vi "FileExplorerMain.vi"(0 "Top Level Folder Path":path, 4 "Tree":string[](tree), 5 "Search Bar":string, 7 "Copy":bool, 9 "Expand / Colapse":bool, 11 "error in (no error)":errorcluster) -> (6 "Report String":string, 15 "error out":errorcluster)   [LabVIEW 2023]
doc: "This VI is the demonstration of the File explorer using tree with options like search, copy, expand/collapse the tree items populated from the input file path."
uses:
  TypeDefs/FileExplorerQueueOperations.ctl
  TypeDefs/FileExplorerStateDataCluster.ctl
  TypeDefs/FileExplorerDataCluster.ctl
panel:
  # "INSTRUCTIONS\n\n1. Run the VI.\n2. Choose the any folder path using \"Top Level Folder Path\" Control.\n3. Tree is populated with the selected folder hierarchy.\n4. Press \"Expand/Collapse\" button to expand or collapse the Folders in the tree.\n5. Enter folder name in the \"Search Bar\" and press enter to expand on particular folder.\n6. Select any files in the tree and press \"Copy\" to copy the file to the desired location.\n7. Whenever a folder is expanded, particular folder details is indicated in the \"Report String\"\n8. Press the Column Headers to sort the tree based on the selection like Date Modified, Type or size"
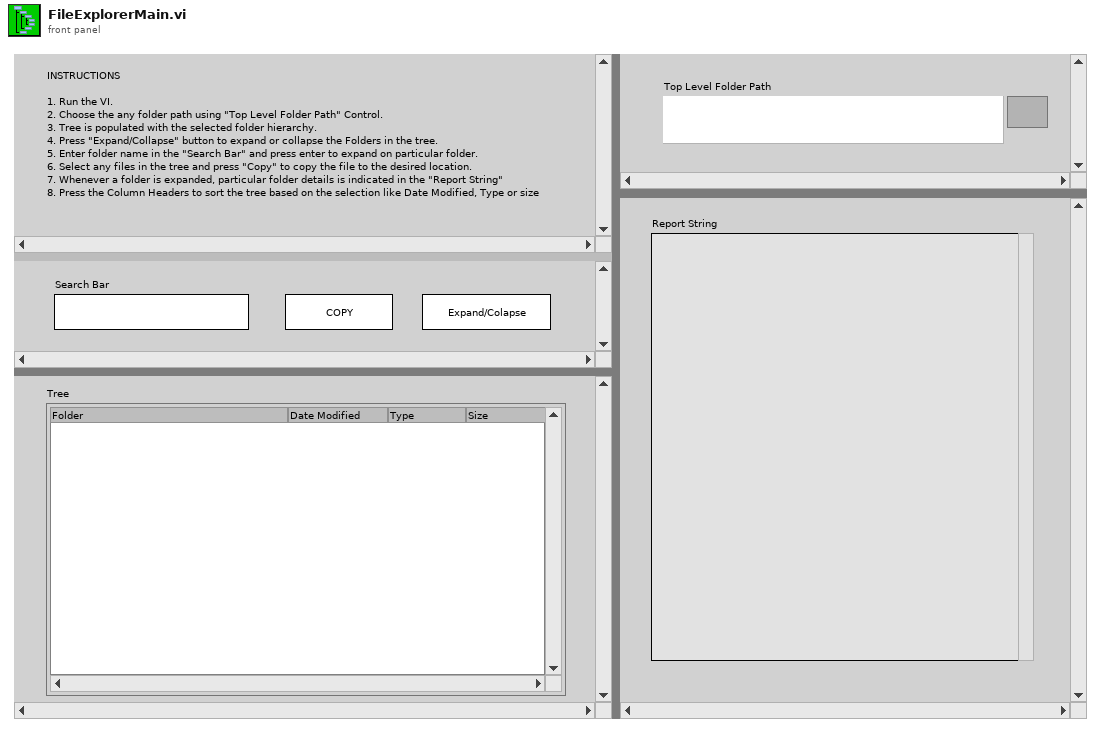
[diagram p1: front panel]
types:
  T1 = typedef "FileExplorerDataCluster.ctl" = cluster{"user event ref":refnum<user-event>, "Search Bar":string, "File Path":path, "All Folders Path":path[], "All Files Path":path[], "Parent Tag":string, "Reverse File Path":path, "End File":string[], "Tag Path":string[], "Selected file array":string[], "Tag Date Modified":string, "Tag Size":string, "Tag Type":string, "Report String":string, "Sort Date":bool, "Sort Type":bool, "Sort Size":bool, "Copied File Path array":path[], "Temp File Path":path, "Copy file Folder":string, "Active Tag":string, "Folders Array":string[]}
  T2 = typedef "FileExplorerStateDataCluster.ctl" = cluster{"State":string, "Data":variant}
  T3 = typedef "FileExplorerQueueOperations.ctl" = enum16{"Init", "Enqueue", "Dequeue", "Enqueue N", "Flush", "Close", "Enqueue N Stack"}
  T4 = typedef "LVPoint32TypeDef.ctl" = cluster{"Horizontal":i32, "Vertical":i32}
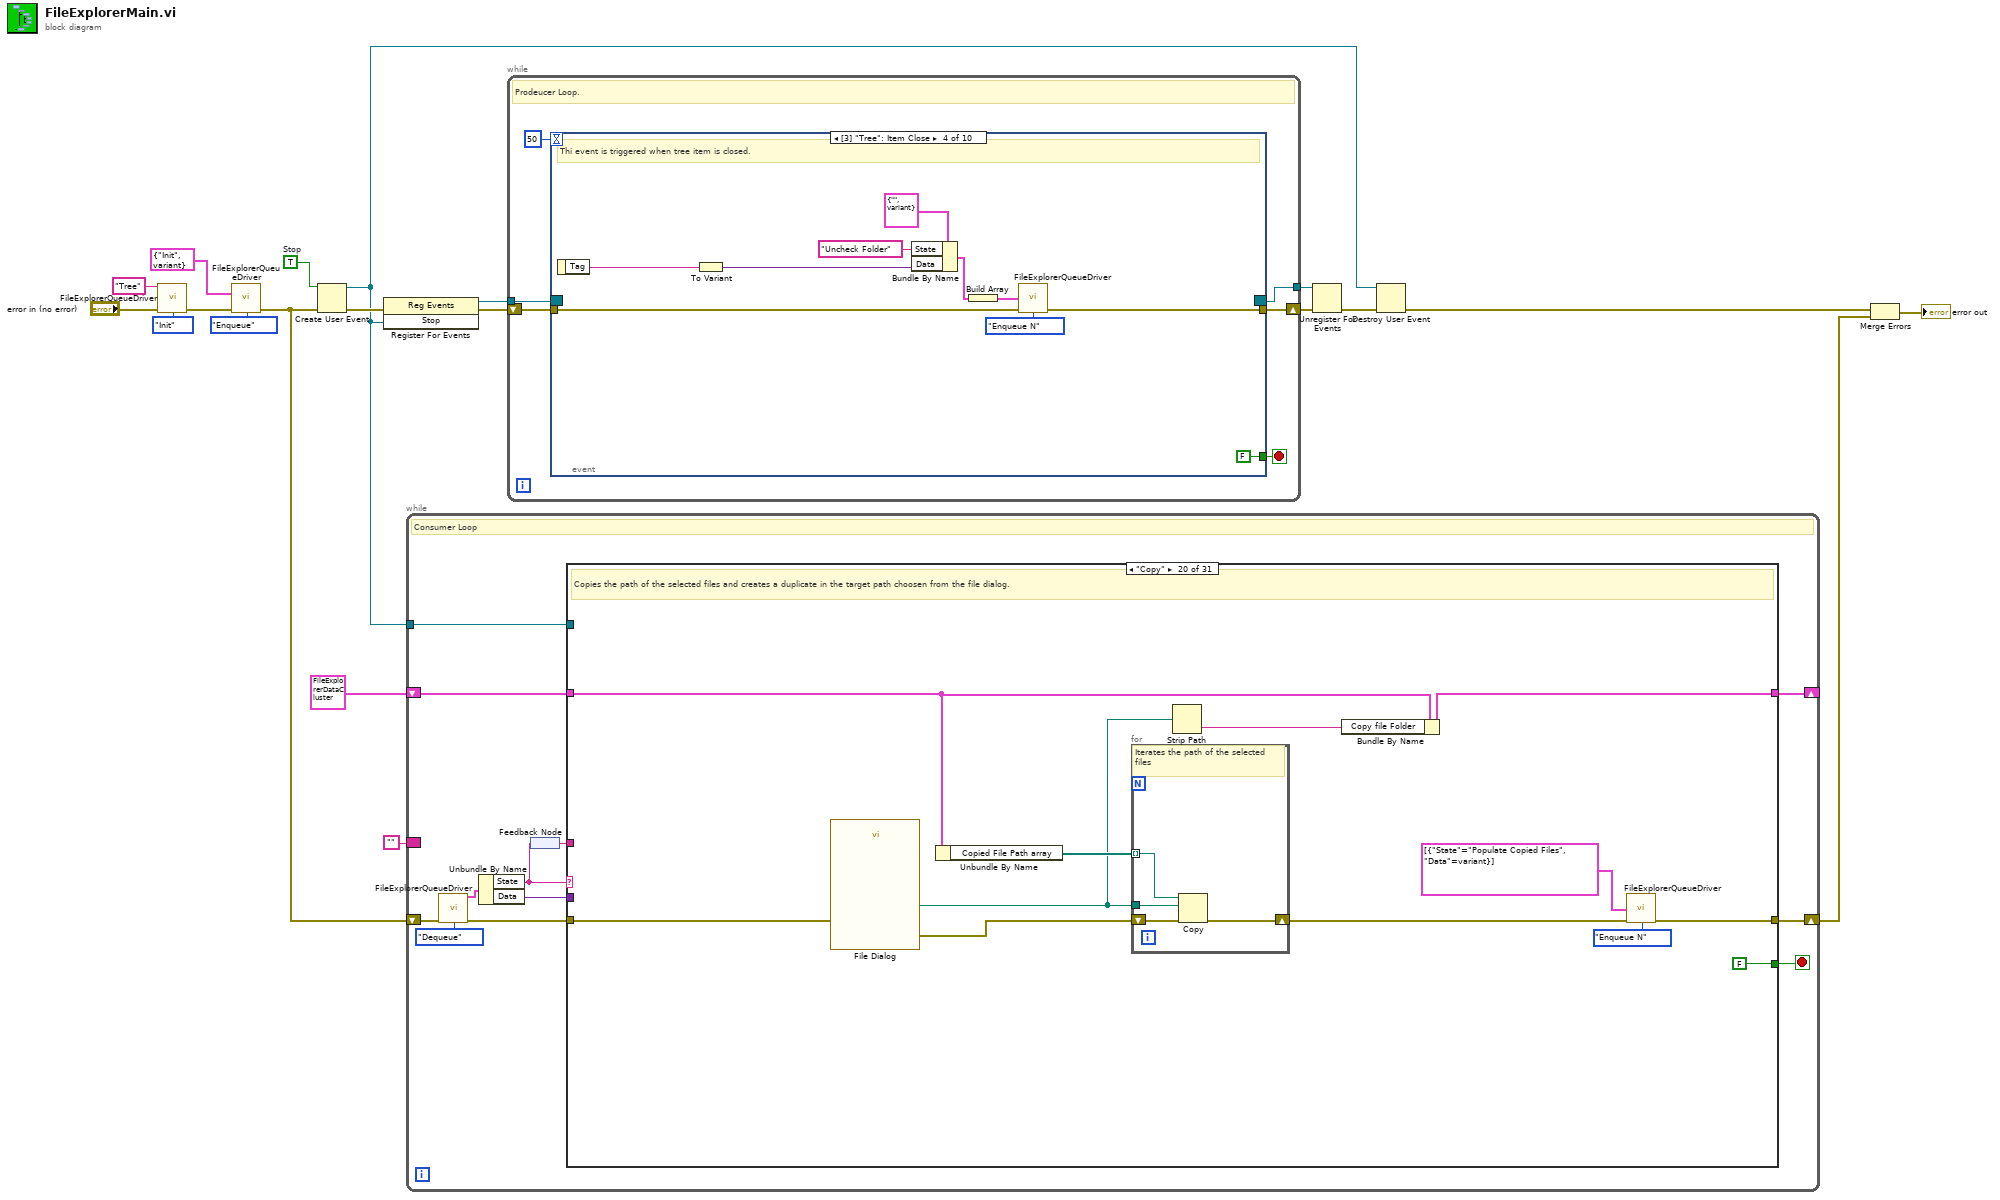
[diagram p0: block diagram]
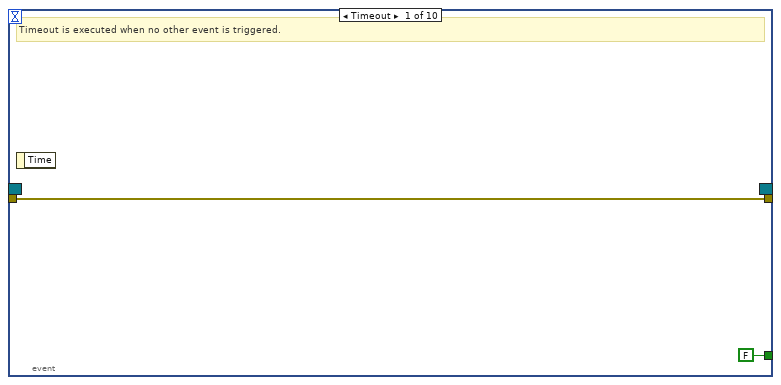
[diagram p2: hidden frame]
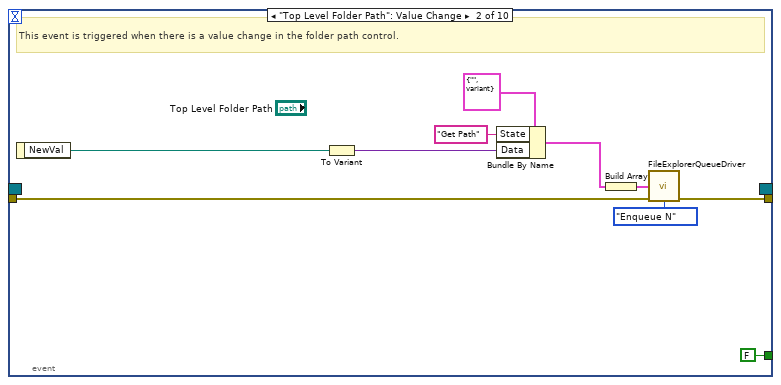
[diagram p3: hidden frame]
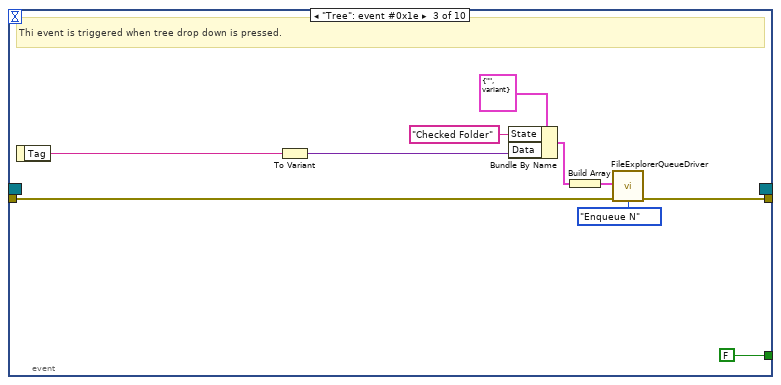
[diagram p4: hidden frame]
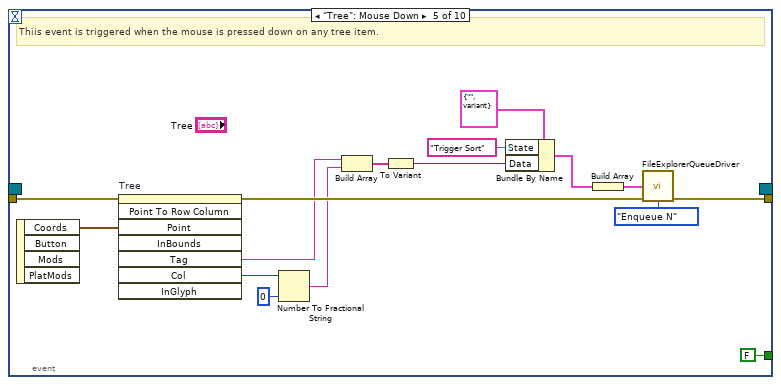
[diagram p5: hidden frame]
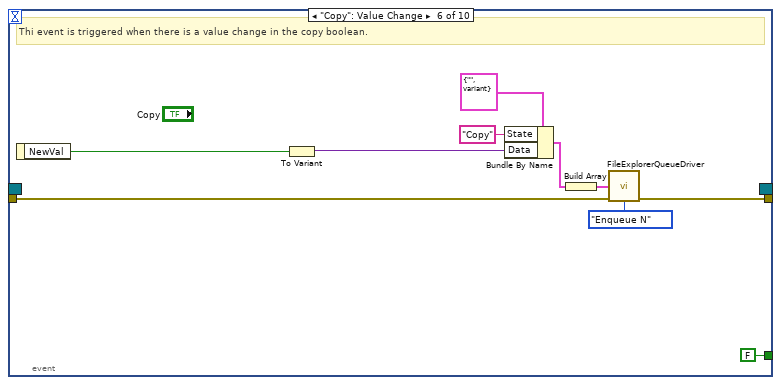
[diagram p6: hidden frame]
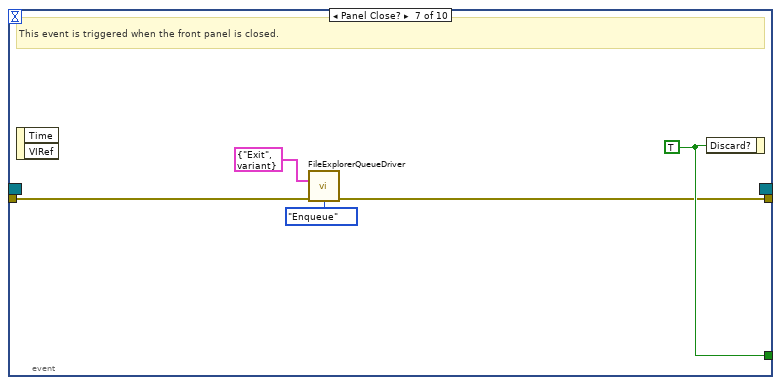
[diagram p7: hidden frame]
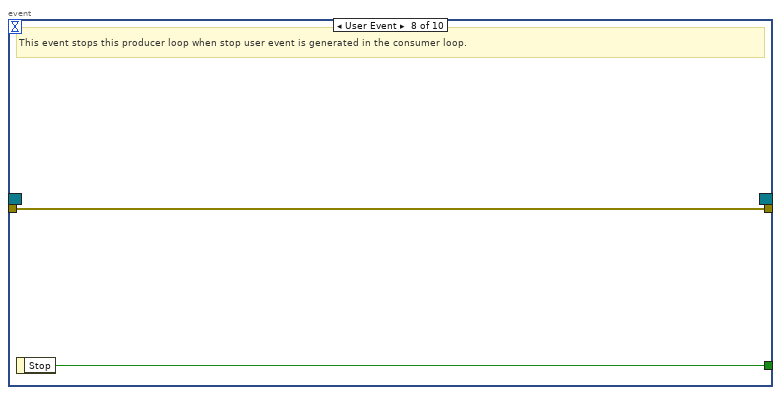
[diagram p8: hidden frame]
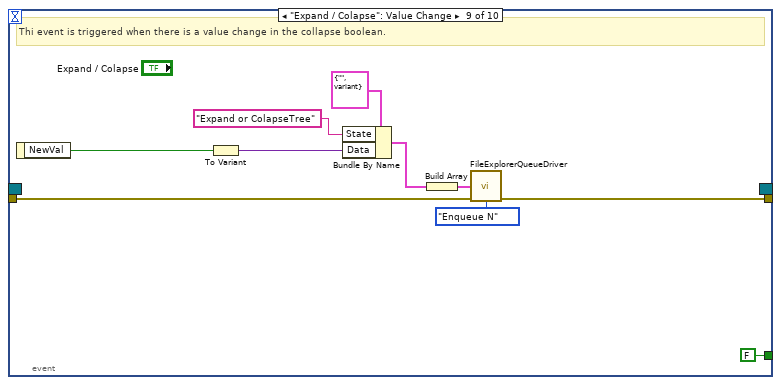
[diagram p9: hidden frame]
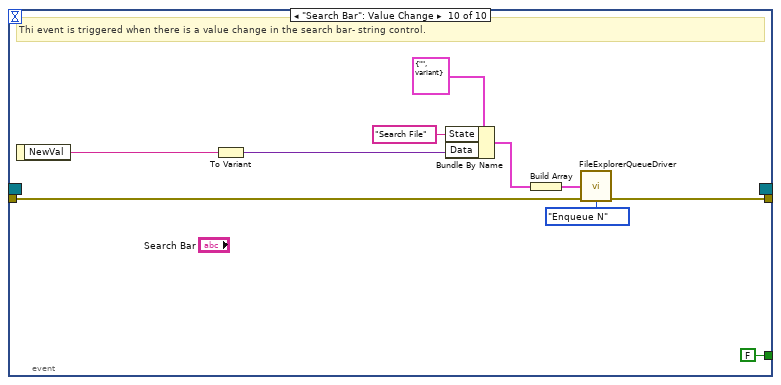
[diagram p10: hidden frame]
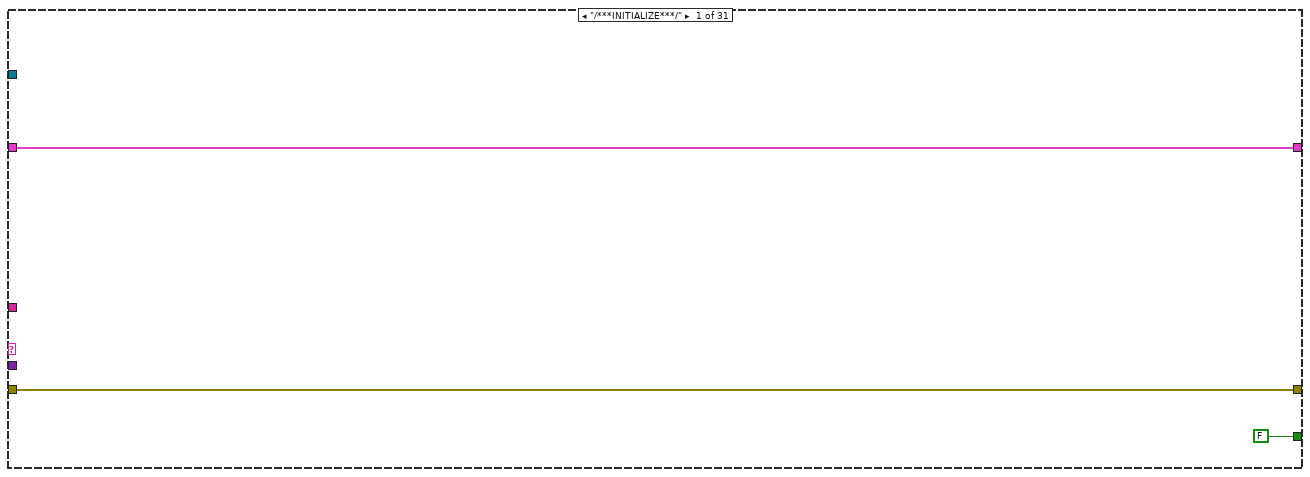
[diagram p11: hidden frame]
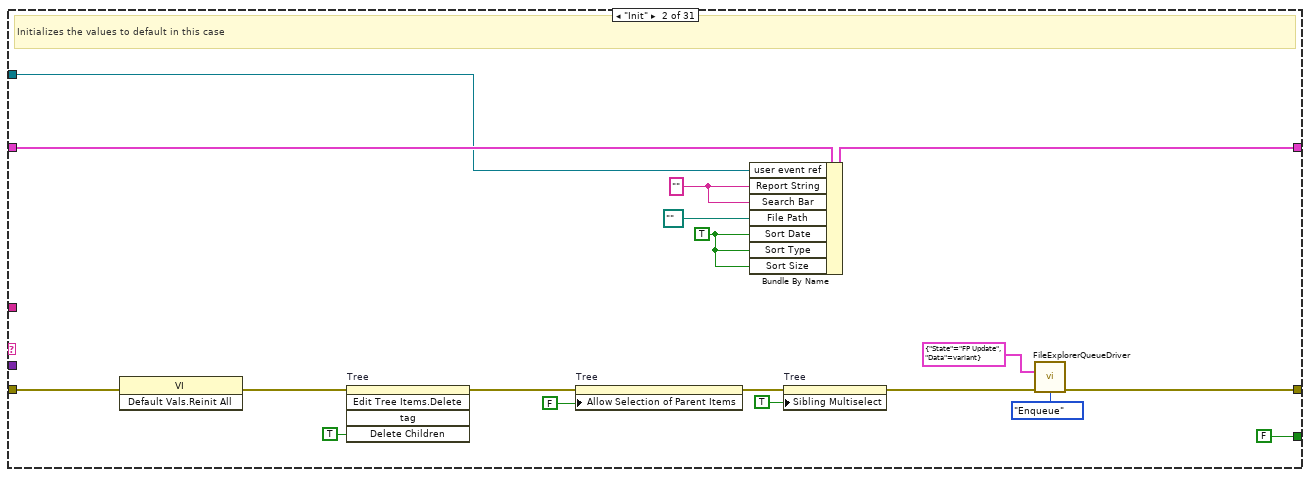
[diagram p12: hidden frame]
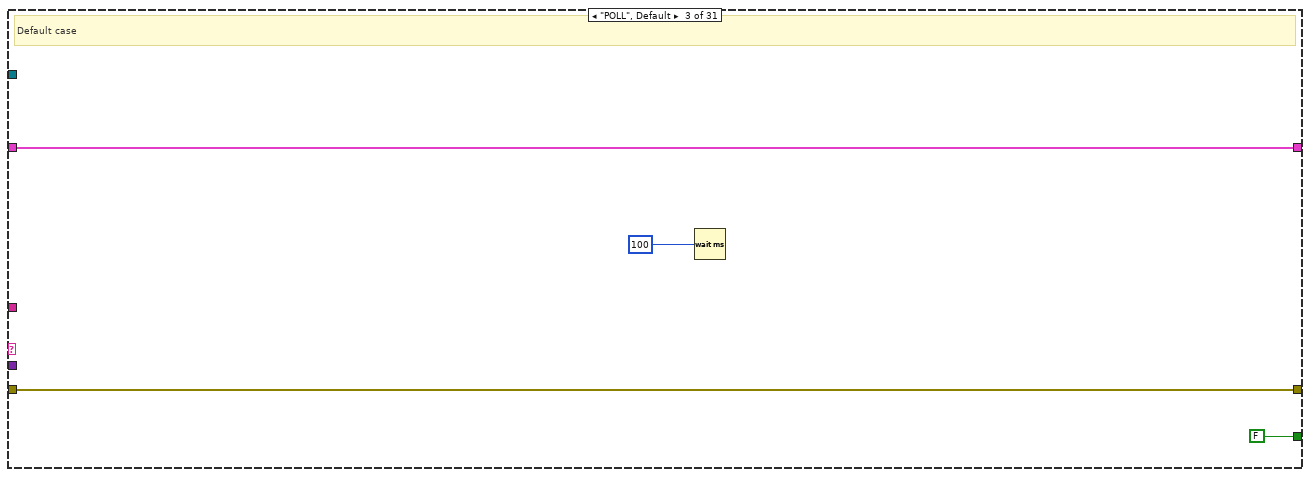
[diagram p13: hidden frame]
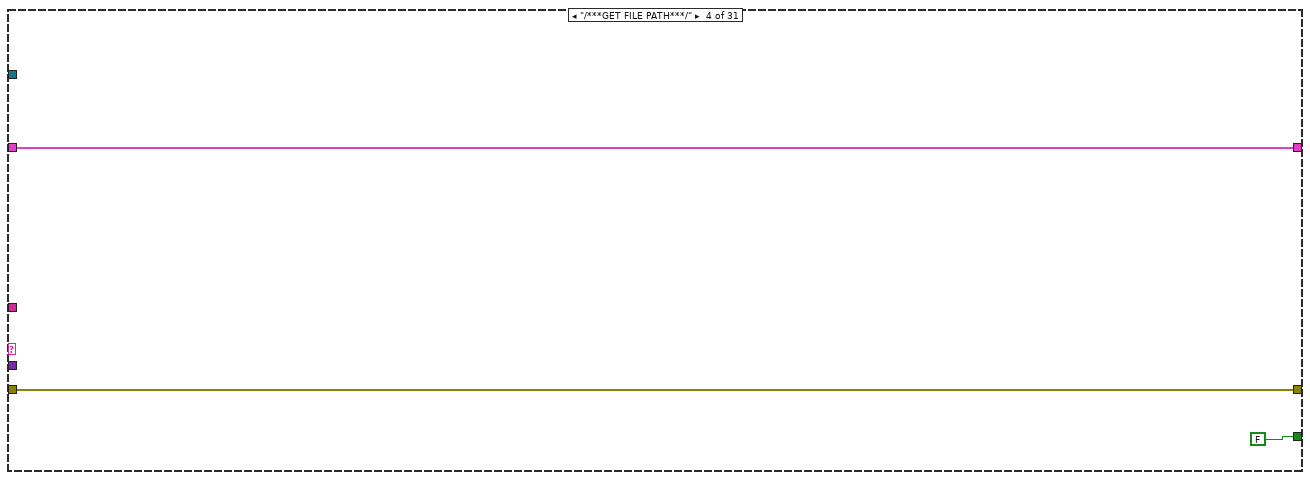
[diagram p14: hidden frame]
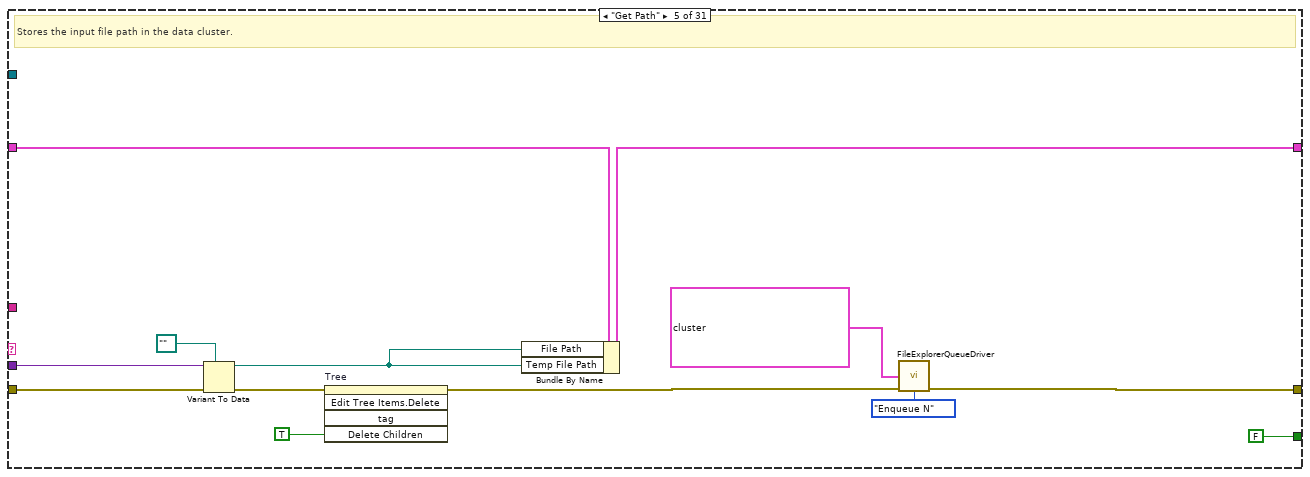
[diagram p15: hidden frame]
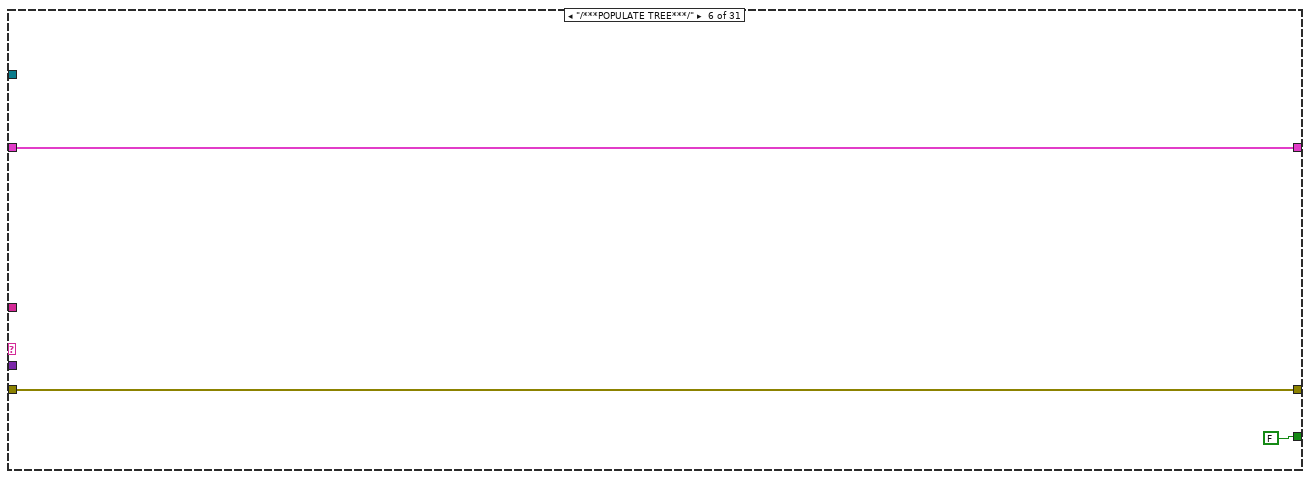
[diagram p16: hidden frame]
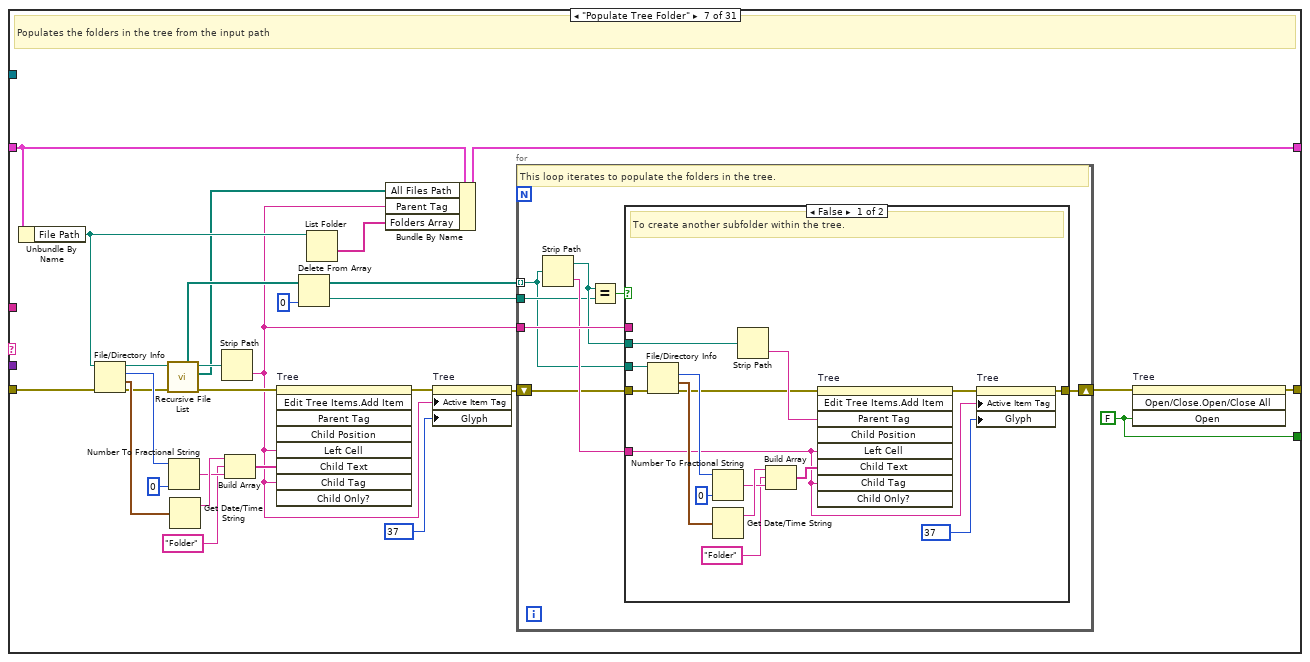
[diagram p17: hidden frame]
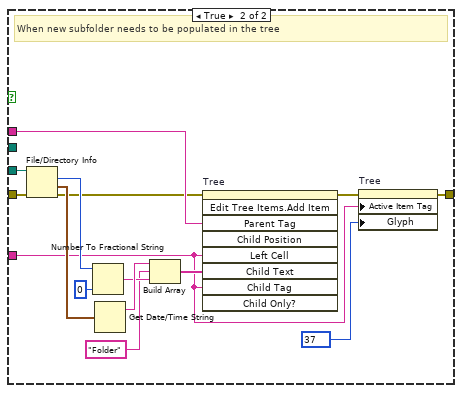
[diagram p18: hidden frame]
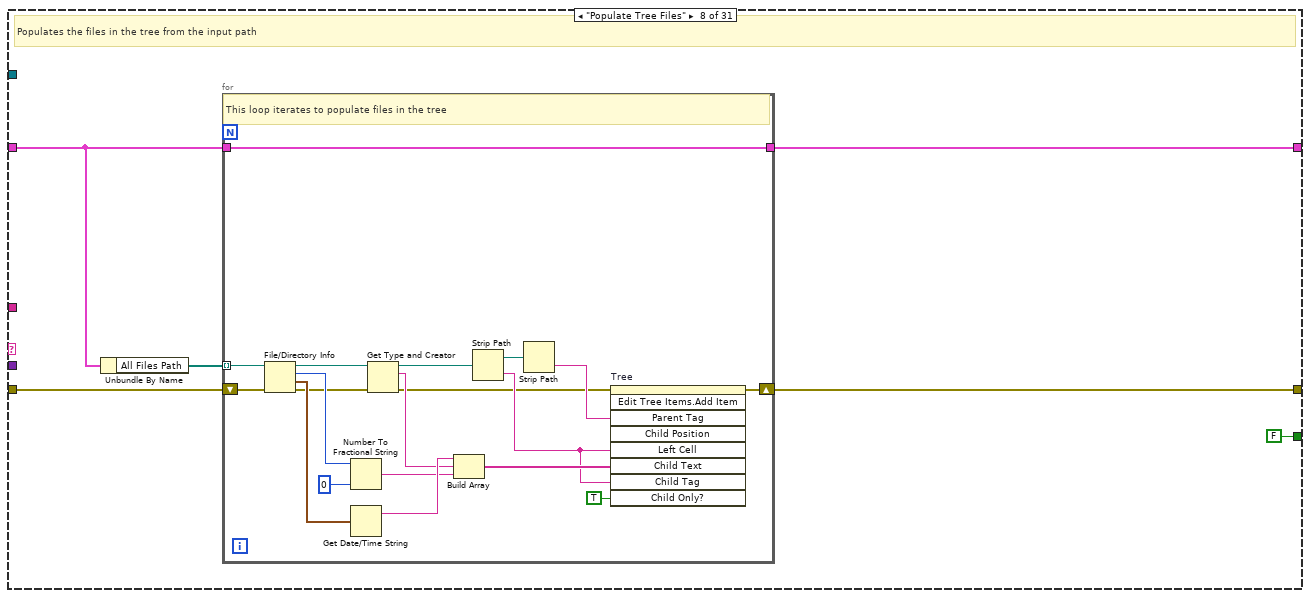
[diagram p19: hidden frame]
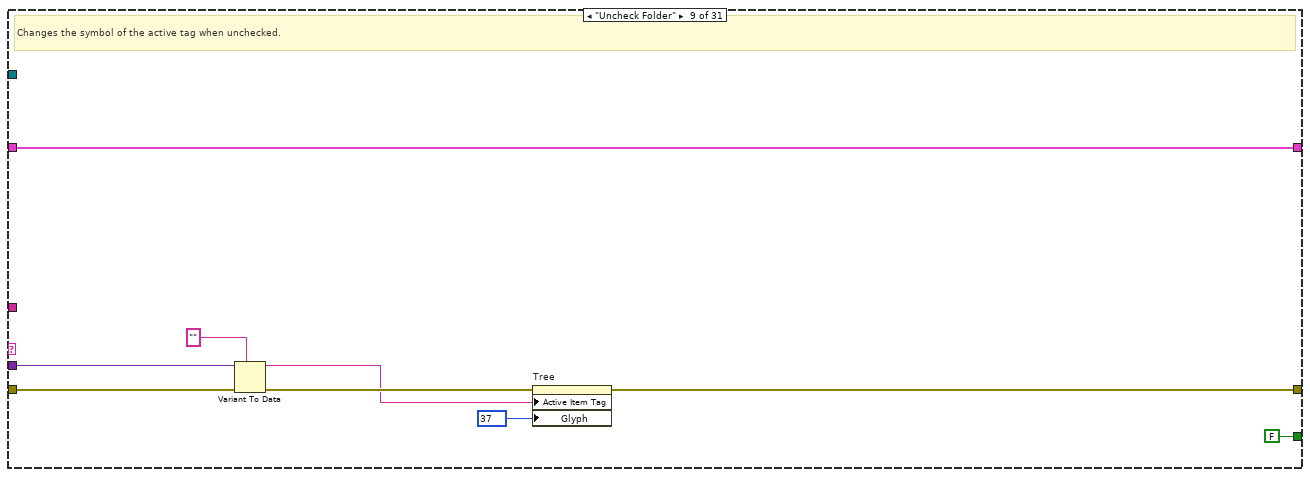
[diagram p20: hidden frame]
diagram:
  w10 = TRUE  # Stop
  n1 = call "FileExplorerQueueDriver.vi"("Queue Name"="Tree", "error in (no error)"="error in (no error)", "Enum"=FileExplorerQueueOperations."Init") -> ("error out"=w13:errorcluster)  [unwired: 11 in, 1 out]
  n2 = call "FileExplorerQueueDriver.vi"("Enqueue Element"=T2 {"State"="Init", "Data"=variant}, "error in (no error)"=w13, "Enum"=FileExplorerQueueOperations."Enqueue") -> ("error out"=w1:errorcluster)  [unwired: 11 in, 1 out]
  n3 = Create User Event(user event datatype=w10, error in=w1) -> (user event=w3:refnum<user-event>, error out=w11:errorcluster)
  n4 = register-events(error in=w11, w3) -> (reference out=w8:refnum<event-registration>, error out=w9:errorcluster)  [unwired: 1 in]
  n5 = while {
    shift-right: [w30] -> w17
    shift-left: w1 -> [w32]
    tunnel: w3 -> [w25]
    shift-right: [w23] -> _
    shift-left: T1 {"user event ref"=refnum, "Search Bar"="", "File Path"=path "", "All Folders Path"=[], "All Files Path"=[], "Parent Tag"="", "Reverse File Path"=path "C:/Users/santha ruban/Desktop/LabVIEW/Batch1", "End File"=[], "Tag Path"=[], "Selected file array"=[], "Tag Date Modified"="", "Tag Size"="", "Tag Type"="", "Report String"="", "Sort Date"=FALSE, "Sort Type"=FALSE, "Sort Size"=FALSE, "Copied File Path array"=[], "Temp File Path"=path "", "Copy file Folder"="", "Active Tag"="", "Folders Array"=[]} -> [w24]
    border: "" ("State") -> [_]
    stop <- w28 stop-if-true
    # "Consumer Loop"
    n6 = call "FileExplorerQueueDriver.vi"("error in (no error)"=w32, "Enum"=FileExplorerQueueOperations."Dequeue") -> ("Dequeue Element"=w27:T2, "error out"=w31:errorcluster)  [unwired: 12 in]
    n7 = Unbundle By Name(w27) -> ("State"=w22:string, "Data"=w26:variant)
    n8 = feedback-in #1(w22) -> ()
    n9 = feedback #1() -> (w21:string)
    n10 = case shown="\"Copy\"" w22 {
      tunnel: w31 -> [w34 w47 w57 w59 w70 w75 w83 w146 w177 w201 w203 w229 w244 w276 w306 w341 w352 w358 w384 w388 w412 w445 w461 w474 w490 w502 w504 w509 w511 w524 w545]
      tunnel: [w34 w44 w57 w59 w69 w75 w90 w145 w176 w184 w215 w229 w232 w272 w302 w340 w351 w354 w384 w390 w406 w444 w461 w468 w490 w494 w504 w509 w511 w530 w543] -> w30
      tunnel: [FALSE FALSE FALSE FALSE FALSE FALSE w84 FALSE FALSE FALSE FALSE FALSE FALSE FALSE FALSE FALSE FALSE FALSE FALSE FALSE FALSE FALSE FALSE FALSE FALSE FALSE FALSE FALSE FALSE FALSE TRUE] -> w28
      tunnel: w26 -> [_ _ _ _ w68 _ _ _ w172 w198 _ _ w243 _ _ w333 w344 _ _ _ w411 _ _ w472 _ w499 _ _ _ _ _]
      tunnel: w25 -> [_ w50 _ _ _ _ _ _ _ _ _ _ _ _ _ _ _ _ _ _ _ _ _ _ _ _ _ _ _ _ _]
      tunnel: w24 -> [w35 w52 w56 w60 w73 w76 w100 w149 w175 w200 w227 w230 w242 w274 w304 w337 w348 w356 w385 w397 w409 w443 w462 w466 w491 w501 w505 w508 w512 w529 w546]
      tunnel: [w35 w51 w56 w60 w72 w76 w99 w148 w175 w197 w219 w230 w241 w273 w303 w337 w348 w355 w385 w395 w408 w442 w462 w466 w491 w501 w505 w508 w512 w527 w546] -> w23
      tunnel: w21 -> [_ _ _ _ _ _ _ _ _ _ _ _ _ _ _ _ _ _ _ _ _ _ _ _ _ _ _ _ _ w521 _]
      frame "/***INITIALIZE***/" {
      }
      frame "Init" {
        w43 = TRUE ("Trigger Sort")
        w46 = "" ("Report String")
        # "Initializes the values to default in this case"
        n11 = invoke class="VI" method="Default Vals.Reinit All"(error in=w47) -> (error out=w40:errorcluster)  [unwired: 2 in, 2 out]
        n12 = invoke on="Tree" class="Tree (strict)" method="Edit Tree Items.Delete"(error in=w40, "Delete Children"=TRUE ("Delete Children?")) -> (error out=w37:errorcluster)  [unwired: 3 in, 4 out]
        n13 = property on="Tree" class="Tree (strict)"(error in=w37, "Allow Selection of Parent Items"=FALSE ("Sibling Multiselect")) -> (error out=w39:errorcluster)  [unwired: 1 in, 1 out]
        n14 = Bundle By Name(cluster=w52, "user event ref"=w50, "Report String"=w46, "Search Bar"=w46, "File Path"=path "", "Sort Date"=w43, "Sort Type"=w43, "Sort Size"=w43) -> (w51:T1)
        n15 = property on="Tree" class="Tree (strict)"(error in=w39, "Sibling Multiselect"=TRUE) -> (error out=w38:errorcluster)  [unwired: 1 in, 1 out]
        n16 = call "FileExplorerQueueDriver.vi"("Enqueue Element"=T2 {"State"="FP Update", "Data"=variant}, "error in (no error)"=w38, "Enum"=FileExplorerQueueOperations."Enqueue") -> ("error out"=w44:errorcluster)  [unwired: 11 in, 1 out]
      }
      frame "POLL", Default {
        # "Default case"
        n17 = Wait (ms)(milliseconds to wait=u32 100) -> ()  [unwired: 1 out]
      }
      frame "/***GET FILE PATH***/" {
      }
      frame "Get Path" {
        # "Stores the input file path in the data cluster."
        n18 = Variant To Data(error in=w70, type=path "" ("NewVal"), Variant=w68) -> (data=w62:path, error out=w64:errorcluster)
        n19 = invoke on="Tree" class="Tree (strict)" method="Edit Tree Items.Delete"(error in=w64, "Delete Children"=TRUE ("Delete Children?")) -> (error out=w63:errorcluster)  [unwired: 3 in, 4 out]
        n20 = Bundle By Name(cluster=w73, "File Path"=w62, "Temp File Path"=w62) -> (w72:T1)
        n21 = call "FileExplorerQueueDriver.vi"("Enqueue N Element"=T2[] [{"State"="Populate Tree Folder", "Data"=variant}, {"State"="Populate Tree Files", "Data"=variant}], "error in (no error)"=w63, "Enum"=FileExplorerQueueOperations."Enqueue N") -> ("error out"=w69:errorcluster)  [unwired: 11 in, 1 out]
      }
      frame "/***POPULATE TREE***/" {
      }
      frame "Populate Tree Folder" {
        w84 = FALSE ("Open?")
        # "Populates the folders in the tree from the input path"
        n22 = Unbundle By Name(w100) -> ("File Path"=w86:path)
        n23 = File/Directory Info(path=w86, error in=w83) -> (path out=w81:path, size=w96:i64, last mod=w98:timestamp, error out=w82:errorcluster)  [unwired: 3 out]
        n24 = call <vilib>:"Recursive File List.vi"("error in (no error)"=w82, "Folder Path"=w81) -> ("error out"=w80:errorcluster, "All Files in Dir"=w78:path[], "dup Folder Path"=w79:path, "All Folders"=w103:path[])  [unwired: 5 in, 1 out]
        n25 = Number To Fractional String(number=w96, precision (6)=i16 0) -> (F-format string=w95:string)  [unwired: 2 in]
        n26 = Get Date/Time String(seconds (now)=w98) -> (date string=w97:string)  [unwired: 2 in, 1 out]
        n27 = Strip Path(path=w79) -> (name=w77:string)  [unwired: 1 out]
        n28 = Build Array(w97, "Folder" ("element"), w95) -> (w92:string[])
        n29 = invoke on="Tree" class="Tree (strict)" method="Edit Tree Items.Add Item"(error in=w80, "Left Cell"=w77, "Child Text"=w92, "Child Tag"=w77) -> (error out=w89:errorcluster)  [unwired: 5 in, 8 out]
        n30 = Delete From Array(array=w103, index=0) -> (deleted portion=w101:path, array with subset deleted=w102:path[])  [unwired: 1 in]
        n31 = List Folder(path=w86) -> (folder names=w85:string[])  [unwired: 3 in, 3 out]
        n32 = Bundle By Name(cluster=w100, "All Files Path"=w78, "Parent Tag"=w77, "Folders Array"=w85) -> (w99:T1)
        n33 = property on="Tree" class="Tree (strict)"(error in=w89, "Active Item Tag"=w77, "Glyph"=37) -> (error out=w88:errorcluster)  [unwired: 1 in, 1 out]
        n34 = for {
          tunnel: w102 -> [w105] mode=indexing
          tunnel: w77 -> [w112]
          tunnel: w101 -> [w106]
          shift-right: [w107] -> w91
          shift-left: w88 -> [w108]
          # "This loop iterates to populate the folders in the tree."
          n35 = Strip Path(path=w105) -> (stripped path=w109:path, name=w111:string)
          n36 = Equal?(x=w109, y=w106) -> (x = y?=w110:bool)
          n37 = case shown="False" w110 {
            tunnel: w112 -> [_ w143]
            tunnel: w111 -> [w115 w132]
            tunnel: w109 -> [w121 _]
            tunnel: w108 -> [w114 w130]
            tunnel: [w116 w133] -> w107
            tunnel: w105 -> [w119 w135]
            frame False {
              # "To create another subfolder within the tree."
              n38 = File/Directory Info(path=w119, error in=w114) -> (size=w125:i64, last mod=w127:timestamp, error out=w113:errorcluster)  [unwired: 4 out]
              n39 = Number To Fractional String(number=w125, precision (6)=i16 0) -> (F-format string=w124:string)  [unwired: 2 in]
              n40 = Get Date/Time String(seconds (now)=w127) -> (date string=w126:string)  [unwired: 2 in, 1 out]
              n41 = Strip Path(path=w121) -> (name=w128:string)  [unwired: 1 out]
              n42 = Build Array(w126, "Folder" ("element"), w124) -> (w122:string[])
              n43 = invoke on="Tree" class="Tree (strict)" method="Edit Tree Items.Add Item"(error in=w113, "Parent Tag"=w128, "Left Cell"=w115, "Child Text"=w122, "Child Tag"=w115) -> (error out=w117:errorcluster)  [unwired: 4 in, 8 out]
              n44 = property on="Tree" class="Tree (strict)"(error in=w117, "Active Item Tag"=w115, "Glyph"=37 ("Active Item:Symbol Index")) -> (error out=w116:errorcluster)  [unwired: 1 in, 1 out]
            }
            frame True {
              # "When new subfolder needs to be populated in the tree"
              n45 = File/Directory Info(path=w135, error in=w130) -> (size=w140:i64, last mod=w142:timestamp, error out=w129:errorcluster)  [unwired: 4 out]
              n46 = Number To Fractional String(number=w140, precision (6)=i16 0) -> (F-format string=w139:string)  [unwired: 2 in]
              n47 = Get Date/Time String(seconds (now)=w142) -> (date string=w141:string)  [unwired: 2 in, 1 out]
              n48 = Build Array(w141, "Folder" ("element"), w139) -> (w137:string[])
              n49 = invoke on="Tree" class="Tree (strict)" method="Edit Tree Items.Add Item"(error in=w129, "Parent Tag"=w143, "Left Cell"=w132, "Child Text"=w137, "Child Tag"=w132) -> (error out=w134:errorcluster)  [unwired: 4 in, 8 out]
              n50 = property on="Tree" class="Tree (strict)"(error in=w134, "Active Item Tag"=w132, "Glyph"=37) -> (error out=w133:errorcluster)  [unwired: 1 in, 1 out]
            }
          }
        }
        n51 = invoke on="Tree" class="Tree (strict)" method="Open/Close.Open/Close All"(error in=w91, "Open"=w84) -> (error out=w90:errorcluster)  [unwired: 2 in, 3 out]
      }
      frame "Populate Tree Files" {
        # "Populates the files in the tree from the input path"
        n52 = Unbundle By Name(w149) -> ("All Files Path"=w147:path[])
        n53 = for {
          tunnel: w149 -> [w168]
          tunnel: [w168] -> w148
          tunnel: w147 -> [w162] mode=indexing
          shift-right: [w167] -> w145
          shift-left: w146 -> [w154]
          # "This loop iterates to populate files in the tree"
          n54 = File/Directory Info(path=w162, error in=w154) -> (path out=w152:path, size=w160:i64, last mod=w164:timestamp, error out=w153:errorcluster)  [unwired: 3 out]
          n55 = Number To Fractional String(number=w160, precision (6)=i16 0) -> (F-format string=w159:string)  [unwired: 2 in]
          n56 = Get Date/Time String(seconds (now)=w164) -> (date string=w163:string)  [unwired: 2 in, 1 out]
          n57 = Get Type and Creator(4:w153, 7:w152) -> (0:w151:errorcluster, 2:w161:string, 3:w150:path)  [unwired: 1 out]
          n58 = Build Array(w163, w161, w159) -> (w158:string[])
          n59 = Strip Path(path=w150) -> (stripped path=w166:path, name=w156:string)
          n60 = Strip Path(path=w166) -> (name=w165:string)  [unwired: 1 out]
          n61 = invoke on="Tree" class="Tree (strict)" method="Edit Tree Items.Add Item"(error in=w151, "Parent Tag"=w165, "Left Cell"=w156, "Child Text"=w158, "Child Tag"=w156, "Child Only?"=TRUE) -> (error out=w167:errorcluster)  [unwired: 3 in, 8 out]
        }
      }
      frame "Uncheck Folder" {
        # "Changes the symbol of the active tag when unchecked."
        n62 = Variant To Data(error in=w177, type="", Variant=w172) -> (data=w170:string, error out=w173:errorcluster)
        n63 = property on="Tree" class="Tree (strict)"(error in=w173, "Active Item Tag"=w170, "Glyph"=37) -> (error out=w176:errorcluster)  [unwired: 1 in, 1 out]
      }
      frame "Checked Folder" {
        # "Changes the symbol of the active tag when checked."
        n64 = Variant To Data(error in=w201, type="" ("Tag"), Variant=w198) -> (data=w179:string, error out=w192:errorcluster)
        n65 = invoke on="Tree" class="Tree (strict)" method="Navigate Tree.Get Path"(error in=w192, "tag"=w179) -> (error out=w191:errorcluster, "Navigate Tree:Get Path"=w196:string[])  [unwired: 2 in, 2 out]
        n66 = property on="Tree" class="Tree (strict)"(error in=w191, "Active Item Tag"=w179, "ActiveColNum"=1 ("Active Cell:Active Column Number")) -> (error out=w193:errorcluster, "Cell String"=w188:string)  [unwired: 1 in, 1 out]
        n67 = property on="Tree" class="Tree (strict)"(error in=w193, "Active Item Tag"=w179, "ActiveColNum"=2 ("Active Cell:Active Column Number")) -> (error out=w194:errorcluster, "Cell String"=w187:string)  [unwired: 1 in, 1 out]
        n68 = property on="Tree" class="Tree (strict)"(error in=w194, "Active Item Tag"=w179, "ActiveColNum"=3 ("Active Cell:Active Column Number")) -> (error out=w182:errorcluster, "Cell String"=w186:string)  [unwired: 1 in, 1 out]
        n69 = property on="Tree" class="Tree (strict)"(error in=w182, "Active Item Tag"=w179, "Glyph"=38) -> (error out=w181:errorcluster)  [unwired: 1 in, 1 out]
        n70 = Bundle By Name(cluster=w200, "Tag Path"=w196, "Tag Date Modified"=w188, "Tag Type"=w187, "Tag Size"=w186) -> (w197:T1)
        n71 = call "FileExplorerQueueDriver.vi"("Enqueue Element"=T2 {"State"="Report Generation", "Data"=variant}, "error in (no error)"=w181, "Enum"=FileExplorerQueueOperations."Enqueue") -> ("error out"=w184:errorcluster)  [unwired: 11 in, 1 out]
      }
      frame "Report Generation" {
        # "Generates report for the active tag of the folder that is checked."
        n72 = Unbundle By Name(w227) -> ("File Path"=w209:path, "Tag Path"=w221:string[], "Tag Date Modified"=w225:string, "Tag Size"=w224:string, "Tag Type"=w223:string, "Report String"=w222:string)
        n73 = Array of Strings to Path(0:w221) -> (2:w207:path)  [unwired: 1 in]
        n74 = Strip Path(path=w209) -> (stripped path=w206:path)  [unwired: 1 out]
        n75 = Path To String(path=w206) -> (string=w220:string)
        n76 = Path To String(path=w207) -> (string=w205:string)
        n77 = Concatenate Strings(w220, "\\" ("string"), w205) -> (w208:string)
        n78 = Format Into String(format string="Path : %s \nLast Modified : %s\nSize : %s \nType : %s ", initial string=w222, error in=w203, w208, w225, w224, w223) -> (resulting string=w218:string, error out=w216:errorcluster)
        n79 = Concatenate Strings(w218, "\r\n", "<---------------------------------------------->" ("string"), "\r\n") -> (w213:string)
        n80 = call "FileExplorerQueueDriver.vi"("Enqueue Element"=T2 {"State"="FP Update", "Data"=variant}, "error in (no error)"=w216, "Enum"=FileExplorerQueueOperations."Enqueue") -> ("error out"=w215:errorcluster)  [unwired: 11 in, 1 out]
        n81 = Bundle By Name(cluster=w227, "Report String"=w213) -> (w219:T1)
      }
      frame "/***SORT TREE***/" {
      }
      frame "Trigger Sort" {
        # "When any of the column header is clicked for sorting this case is executed."
        n82 = Variant To Data(error in=w244, type=string[] [] ("appended array"), Variant=w243) -> (data=w239:string[], error out=w240:errorcluster)
        n83 = Index Array(array=w239, index #1=0 ("index"), index #2=1 ("index")) -> (element #1=w233:string, element #2=w235:string)
        n84 = Concatenate Strings(w233, w235) -> (w234:string)
        n85 = case shown="\"TREE_COLUMN_HEADERS3\"" w234 {
          tunnel: w242 -> [w249 w260 w265 w270]
          tunnel: [w249 w251 w265 w270] -> w241
          tunnel: w240 -> [w247 w253 w263 w268]
          tunnel: [w246 w252 w262 w267] -> w232
          tunnel: w233 -> [_ w250 _ _]
          frame "TREE_COLUMN_HEADERS1" {
            # "When Date modified is clicked to sort the tree."
            n86 = call "FileExplorerQueueDriver.vi"("Enqueue Element"=T2 {"State"="Sort by Date Modified", "Data"=variant}, "error in (no error)"=w247, "Enum"=FileExplorerQueueOperations."Enqueue") -> ("error out"=w246:errorcluster)  [unwired: 11 in, 1 out]
          }
          frame Default {
            # "When the column header is not clicked."
            n87 = To Variant(anything=w250) -> (Variant=w254:variant)
            n88 = Bundle By Name(cluster=w260, "Active Tag"=w250) -> (w251:T1)
            n89 = Bundle By Name(cluster=T2 {"State"="", "Data"=variant} ("Dequeue Element"), "State"="Selected Files", "Data"=w254) -> (w256:T2)
            n90 = Build Array(w256) -> (w255:T2[])
            n91 = call "FileExplorerQueueDriver.vi"("Enqueue N Element"=w255, "error in (no error)"=w253, "Enum"=FileExplorerQueueOperations."Enqueue N") -> ("error out"=w252:errorcluster)  [unwired: 11 in, 1 out]
          }
          frame "TREE_COLUMN_HEADERS3" {
            # "When size is clicked to sort the tree."
            n92 = call "FileExplorerQueueDriver.vi"("Enqueue Element"=T2 {"State"="Sort by Size", "Data"=variant}, "error in (no error)"=w263, "Enum"=FileExplorerQueueOperations."Enqueue") -> ("error out"=w262:errorcluster)  [unwired: 11 in, 1 out]
          }
          frame "TREE_COLUMN_HEADERS2" {
            # "When Type is clicked to sort the tree."
            n93 = call "FileExplorerQueueDriver.vi"("Enqueue Element"=T2 {"State"="Sort by Type", "Data"=variant}, "error in (no error)"=w268, "Enum"=FileExplorerQueueOperations."Enqueue") -> ("error out"=w267:errorcluster)  [unwired: 11 in, 1 out]
          }
        }
      }
      frame "Sort by Date Modified" {
        # "When Date modified header is clicked the tree is sorted by the date modified."
        n94 = Unbundle By Name(w274) -> ("Sort Date"=w275:bool)
        n95 = case shown="False" w275 {
          tunnel: w274 -> [w288 w300]
          tunnel: [w287 w299] -> w273
          tunnel: w276 -> [w280 w292]
          tunnel: [w279 w291] -> w272
          frame False {
            # "When Date modified is clicked for the second time"
            n96 = To Variant(anything=1) -> (Variant=w277:variant)
            n97 = Bundle By Name(cluster=T2 {"State"="", "Data"=variant} ("Dequeue Element"), "State"="Sort Tree Descending", "Data"=w277) -> (w282:T2)
            n98 = Bundle By Name(cluster=w288, "Sort Date"=TRUE ("Trigger Sort")) -> (w287:T1)
            n99 = Build Array(w282) -> (w281:T2[])
            n100 = call "FileExplorerQueueDriver.vi"("Enqueue N Element"=w281, "error in (no error)"=w280, "Enum"=FileExplorerQueueOperations."Enqueue N") -> ("error out"=w279:errorcluster)  [unwired: 11 in, 1 out]
          }
          frame True {
            # "When Date modified is clicked once"
            n101 = To Variant(anything=1) -> (Variant=w289:variant)
            n102 = Bundle By Name(cluster=T2 {"State"="", "Data"=variant} ("Dequeue Element"), "State"="Sort Tree Ascending", "Data"=w289) -> (w294:T2)
            n103 = Bundle By Name(cluster=w300, "Sort Date"=FALSE ("Trigger Sort")) -> (w299:T1)
            n104 = Build Array(w294) -> (w293:T2[])
            n105 = call "FileExplorerQueueDriver.vi"("Enqueue N Element"=w293, "error in (no error)"=w292, "Enum"=FileExplorerQueueOperations."Enqueue N") -> ("error out"=w291:errorcluster)  [unwired: 11 in, 1 out]
          }
        }
      }
      frame "Sort by Type" {
        # "When Type header is clicked the tree is sorted by the Type order."
        n106 = Unbundle By Name(w304) -> ("Sort Type"=w305:bool)
        n107 = case shown="False" w305 {
          tunnel: w304 -> [w318 w330]
          tunnel: [w317 w329] -> w303
          tunnel: w306 -> [w310 w322]
          tunnel: [w309 w321] -> w302
          frame False {
            # "When Type is clicked for the second time"
            n108 = To Variant(anything=2) -> (Variant=w307:variant)
            n109 = Bundle By Name(cluster=T2 {"State"="", "Data"=variant} ("Dequeue Element"), "State"="Sort Tree Descending", "Data"=w307) -> (w312:T2)
            n110 = Bundle By Name(cluster=w318, "Sort Type"=TRUE ("Trigger Sort")) -> (w317:T1)
            n111 = Build Array(w312) -> (w311:T2[])
            n112 = call "FileExplorerQueueDriver.vi"("Enqueue N Element"=w311, "error in (no error)"=w310, "Enum"=FileExplorerQueueOperations."Enqueue N") -> ("error out"=w309:errorcluster)  [unwired: 11 in, 1 out]
          }
          frame True {
            # "When type is clicked for the second time"
            n113 = To Variant(anything=2) -> (Variant=w319:variant)
            n114 = Bundle By Name(cluster=T2 {"State"="", "Data"=variant} ("Dequeue Element"), "State"="Sort Tree Ascending", "Data"=w319) -> (w324:T2)
            n115 = Bundle By Name(cluster=w330, "Sort Type"=FALSE ("Trigger Sort")) -> (w329:T1)
            n116 = Build Array(w324) -> (w323:T2[])
            n117 = call "FileExplorerQueueDriver.vi"("Enqueue N Element"=w323, "error in (no error)"=w322, "Enum"=FileExplorerQueueOperations."Enqueue N") -> ("error out"=w321:errorcluster)  [unwired: 11 in, 1 out]
          }
        }
      }
      frame "Sort Tree Ascending" {
        # "Sorts the tree in ascending order when clicked once"
        n118 = Variant To Data(error in=w341, type=1 ("Sort Column"), Variant=w333) -> (data=w332:i32, error out=w335:errorcluster)
        n119 = Unbundle By Name(w337) -> ("Parent Tag"=w336:string)
        n120 = invoke on="Tree" class="Tree (strict)" method="Edit Tree Items.Sort Children"(error in=w335, "tag"=w336, "Sort Column"=w332, "Sort Recursively"=TRUE ("Sort Recursively?"), "Reverse Order"=FALSE ("Reverse Order?")) -> (error out=w340:errorcluster)  [unwired: 3 in, 7 out]
      }
      frame "Sort Tree Descending" {
        # "Sorts the tree in descending order when clicked for the second time."
        n121 = Variant To Data(error in=w352, type=1 ("Sort Column"), Variant=w344) -> (data=w343:i32, error out=w346:errorcluster)
        n122 = Unbundle By Name(w348) -> ("Parent Tag"=w347:string)
        n123 = invoke on="Tree" class="Tree (strict)" method="Edit Tree Items.Sort Children"(error in=w346, "tag"=w347, "Sort Column"=w343, "Sort Recursively"=TRUE ("Sort Recursively?"), "Reverse Order"=TRUE ("Reverse Order?")) -> (error out=w351:errorcluster)  [unwired: 3 in, 7 out]
      }
      frame "Sort by Size" {
        # "When Size header is clicked the tree is sorted according to the size."
        n124 = Unbundle By Name(w356) -> ("Sort Size"=w357:bool)
        n125 = case shown="False" w357 {
          tunnel: w356 -> [w370 w382]
          tunnel: [w369 w381] -> w355
          tunnel: w358 -> [w362 w374]
          tunnel: [w361 w373] -> w354
          frame False {
            # "When Size is clicked for the second time"
            n126 = To Variant(anything=3) -> (Variant=w359:variant)
            n127 = Bundle By Name(cluster=T2 {"State"="", "Data"=variant} ("Dequeue Element"), "State"="Sort Tree Descending", "Data"=w359) -> (w364:T2)
            n128 = Bundle By Name(cluster=w370, "Sort Size"=TRUE ("Trigger Sort")) -> (w369:T1)
            n129 = Build Array(w364) -> (w363:T2[])
            n130 = call "FileExplorerQueueDriver.vi"("Enqueue N Element"=w363, "error in (no error)"=w362, "Enum"=FileExplorerQueueOperations."Enqueue N") -> ("error out"=w361:errorcluster)  [unwired: 11 in, 1 out]
          }
          frame True {
            # "When Size is clicked once."
            n131 = To Variant(anything=3) -> (Variant=w371:variant)
            n132 = Bundle By Name(cluster=T2 {"State"="", "Data"=variant} ("Dequeue Element"), "State"="Sort Tree Ascending", "Data"=w371) -> (w376:T2)
            n133 = Bundle By Name(cluster=w382, "Sort Size"=FALSE ("Trigger Sort")) -> (w381:T1)
            n134 = Build Array(w376) -> (w375:T2[])
            n135 = call "FileExplorerQueueDriver.vi"("Enqueue N Element"=w375, "error in (no error)"=w374, "Enum"=FileExplorerQueueOperations."Enqueue N") -> ("error out"=w373:errorcluster)  [unwired: 11 in, 1 out]
          }
        }
      }
      frame "/***COPY FILES***/" {
      }
      frame "Copy" {
        # "Copies the path of the selected files and creates a duplicate in the target path choosen from the file dialog."
        n136 = call "File Dialog"("error in"=w388) -> ("selected path"=w394:path, "error out"=w387:errorcluster)  [unwired: 11 in, 2 out]
        n137 = Unbundle By Name(w397) -> ("Copied File Path array"=w396:path[])
        n138 = for {
          tunnel: w394 -> [w398]
          shift-right: [w400] -> w391
          shift-left: w387 -> [w401]
          tunnel: w396 -> [w399] mode=indexing
          # "Iterates the path of the selected files"
          n139 = Copy(8:w401, 10:w398, 11:w399) -> (0:w400:errorcluster)  [unwired: 2 in, 2 out]
        }
        n140 = Strip Path(path=w394) -> (name=w393:string)  [unwired: 1 out]
        n141 = Bundle By Name(cluster=w397, "Copy file Folder"=w393) -> (w395:T1)
        n142 = call "FileExplorerQueueDriver.vi"("Enqueue N Element"=T2[] [{"State"="Populate Copied Files", "Data"=variant}], "error in (no error)"=w391, "Enum"=FileExplorerQueueOperations."Enqueue N") -> ("error out"=w390:errorcluster)  [unwired: 11 in, 1 out]
      }
      frame "Selected Files" {
        # "Selected tree item is check whether a file or folder and when it is a file, selected file is added to an array."
        n143 = Variant To Data(error in=w412, type="" ("Tag"), Variant=w411) -> (data=w402:string, error out=w407:errorcluster)
        n144 = property on="Tree" class="Tree (strict)"(error in=w407, "Active Item Tag"=w402) -> (error out=w405:errorcluster, "Child-Only?"=w404:bool)  [unwired: 1 in, 1 out]
        n145 = case shown="True" w404 {
          tunnel: w409 -> [w414 w429]
          tunnel: [w414 w427] -> w408
          tunnel: [w413 w417] -> w406
          tunnel: w405 -> [w413 w416]
          tunnel: w402 -> [_ w415]
          frame False {
            # "When the selected files are not a child-only file"
          }
          frame True {
            # "When the selected files are child-only files."
            n146 = Unbundle By Name(w429) -> ("Selected file array"=w428:string[], "Temp File Path"=w424:path, "Copied File Path array"=w422:path[])
            n147 = Build Array (concatenate)(w428, w415) -> (w426:string[])
            n148 = invoke on="Tree" class="Tree (strict)" method="Navigate Tree.Get Path"(error in=w416, "tag"=w415) -> (error out=w417:errorcluster, "Navigate Tree:Get Path"=w425:string[])  [unwired: 2 in, 2 out]
            n149 = Array of Strings to Path(0:w425) -> (2:w423:path)  [unwired: 1 in]
            n150 = Strip Path(path=w423) -> (name=w419:string)  [unwired: 1 out]
            n151 = String To Path(string=w419) -> (path=w418:path)
            n152 = Build Path(base path=w424, name or relative path=w418) -> (appended path=w421:path)
            n153 = Build Array (concatenate)(w422, w421) -> (w420:path[])
            n154 = Bundle By Name(cluster=w429, "Selected file array"=w426, "Copied File Path array"=w420) -> (w427:T1)
          }
        }
      }
      frame "Populate Copied Files" {
        # "Added files in the array is then populated in the tree with its corresponding folder."
        n155 = Unbundle By Name(w443) -> ("Selected file array"=w436:string[], "Copy file Folder"=w435:string, "Temp File Path"=w440:path)
        n156 = List Folder(path=w440, error in=w445) -> (folder names=w430:string[], error out=w439:errorcluster)  [unwired: 2 in, 2 out]
        n157 = for {
          tunnel: w436 -> [w458]
          tunnel: [w458] -> w437
          tunnel: w430 -> [w457] mode=indexing
          tunnel: w435 -> [w455]
          tunnel: [w456] -> w434
          tunnel: [w455] -> w433
          shift-right: [w459] -> w438
          shift-left: w439 -> [w459]
          # "Iterates to check the copied folder already exists in the tree."
          n158 = Equal?(x=w455, y=w457) -> (x = y?=w456:bool)
        }
        n159 = Bundle By Name(cluster=w443, "Folders Array"=w430) -> (w431:T1)
        n160 = case shown="True" w434 {
          tunnel: [w446 w450] -> w444
          tunnel: w438 -> [w446 w449]
          tunnel: w437 -> [_ w448]
          tunnel: w433 -> [_ w447]
          frame False {
            # "When the folder path choosen from the file dialog is parallel to the input file path."
          }
          frame True {
            # "When the folder path choosen from the file dialog is parallel to the input file path."
            n161 = for {
              tunnel: w448 -> [w452] mode=indexing
              tunnel: w447 -> [w451]
              shift-right: [w453] -> w450
              shift-left: w449 -> [w454]
              # "Iterates to populate the copied  files in the tree"
              n162 = invoke on="Tree" class="Tree (strict)" method="Edit Tree Items.Add Item"(error in=w454, "Parent Tag"=w451, "Left Cell"=w452) -> (error out=w453:errorcluster)  [unwired: 6 in, 8 out]
            }
          }
        }
        n163 = Bundle By Name(cluster=w431, "Selected file array"=string[] []) -> (w442:T1)
      }
      frame "/***EXPAND COLAPSE TREE***/" {
      }
      frame "Expand or ColapseTree" {
        # "Expands or collapses the tree when pressed."
        n164 = Variant To Data(error in=w474, type=TRUE, Variant=w472) -> (data=w467:bool, error out=w473:errorcluster)
        n165 = invoke on="Tree" class="Tree (strict)" method="Open/Close.Open/Close All"(error in=w473, "Open"=w467) -> (error out=w470:errorcluster)  [unwired: 2 in, 3 out]
        n166 = Unbundle By Name(w466) -> ("Parent Tag"=w465:string, "Folders Array"=w464:string[])
        n167 = Build Array (concatenate)(w465, w464) -> (w463:string[])
        n168 = case shown="True" w467 {
          tunnel: w470 -> [w477 w484]
          tunnel: [w476 w483] -> w468
          tunnel: w463 -> [w475 w482]
          frame True {
            # "When expand all is pressed, checkbox symbol is changed accordingly"
            n169 = for {
              shift-right: [w480] -> w476
              shift-left: w477 -> [w481]
              tunnel: w475 -> [w478] mode=indexing
              # "Folder Array is iterated to get all the tags of the folders"
              n170 = property on="Tree" class="Tree (strict)"(error in=w481, "Active Item Tag"=w478, "Glyph"=38) -> (error out=w480:errorcluster)  [unwired: 1 in, 1 out]
            }
          }
          frame False {
            # "When collapse all is pressed, checkbox symbol is changed accordingly"
            n171 = for {
              shift-right: [w487] -> w483
              shift-left: w484 -> [w488]
              tunnel: w482 -> [w485] mode=indexing
              # "Folder Array is iterated to get all the tags of the folders"
              n172 = property on="Tree" class="Tree (strict)"(error in=w488, "Active Item Tag"=w485, "Glyph"=37) -> (error out=w487:errorcluster)  [unwired: 1 in, 1 out]
            }
          }
        }
      }
      frame "/***SEARCH FILE ***/" {
      }
      frame "Search File" {
        # "Opens the searched file in the tree when it is found."
        n173 = Variant To Data(error in=w502, type="", Variant=w499) -> (data=w493:string, error out=w500:errorcluster)
        n174 = invoke on="Tree" class="Tree (strict)" method="Open/Close.Item"(error in=w500, "tag"=w493, "Open"=TRUE ("Open?")) -> (error out=w497:errorcluster)  [unwired: 2 in, 4 out]
        n175 = property on="Tree" class="Tree (strict)"(error in=w497, "Active Item Tag"=w493, "Glyph"=38) -> (error out=w494:errorcluster)  [unwired: 1 in, 1 out]
      }
      frame "/***FRONT PANEL UPDATE***/" {
      }
      frame "FP Update" {
        # "Updates the front panel indicators."
        n176 = Unbundle By Name(w508) -> ("Report String"=→"Report String":string)
      }
      frame "/***ERROR***/" {
      }
      frame "Error" {
        # "When any error occurs, this state popups the error and state from where the error has occured."
        n177 = Unbundle By Name(w524) -> ("status"=w520:bool, "code"=w519:i32)
        n178 = call <vilib>:"Clear Errors.vi"("error in (no error)"=w524) -> ("error out"=w523:errorcluster)  [unwired: 5 in, 1 out]
        n179 = Format Into String(format string="Erro occured at State : %s \nError Status : %s\nError Code : %d", initial string="", error in=w523, w521, w520, w519) -> (resulting string=w516:string, error out=w522:errorcluster)
        n180 = Two Button Dialog(message=w516, 1:"Exit" ("F button name (\"Cancel\")"), 2:"Continue" ("T button name (\"OK\")")) -> (T button?=w513:bool)
        n181 = Unbundle By Name(w529) -> ("user event ref"=w528:refnum<user-event>)
        n182 = case shown="False" w513 {
          tunnel: [w531 w538] -> w530
          tunnel: w522 -> [w531 w535]
          tunnel: w528 -> [w532 w534]
          tunnel: [w532 w533] -> w526
          frame True {
          }
          frame False {
            # "When user clicks Exit after an error occurs, and when exit is presed VI is aborted"
            n183 = call "FileExplorerQueueDriver.vi"("Enqueue Element"=T2 {"State"="Exit", "Data"=variant}, "error in (no error)"=w535, "Enum"=FileExplorerQueueOperations."Enqueue") -> ("error out"=w539:errorcluster)  [unwired: 11 in, 1 out]
            n184 = Generate User Event(user event=w534, event data cluster=TRUE ("event data"), error in=w539) -> (user event out=w533:refnum<user-event>, error out=w538:errorcluster)  [unwired: 1 in]
          }
        }
        n185 = Bundle By Name(cluster=w529, "user event ref"=w526) -> (w527:T1)
      }
      frame "Exit" {
        # "Exits the consumer loop."
        n186 = call "FileExplorerQueueDriver.vi"("error in (no error)"=w545, "Enum"=FileExplorerQueueOperations."Flush") -> ("error out"=w544:errorcluster)  [unwired: 12 in, 1 out]
        n187 = call "FileExplorerQueueDriver.vi"("error in (no error)"=w544, "Enum"=FileExplorerQueueOperations."Close") -> ("error out"=w543:errorcluster)  [unwired: 12 in, 1 out]
      }
    }
  }
  n188 = while {
    shift-right: [w552] -> w16
    shift-left: w9 -> [w553]
    tunnel: w8 -> [w549]
    tunnel: [w548] -> w6
    stop <- w550 stop-if-true
    # "Prodeucer Loop."
    n189 = event shown="[3] \"Tree\": Item Close" {
      selector: w549 -> [_ _ _ _ _ _ _ _ _ _]
      dyn-events: [_ _ _ _ _ _ _ _ _ _] -> w548
      timeout: 50 -> [_ _ _ _ _ _ _ _ _ _]
      tunnel: w553 -> [w555 w560 w570 w578 w600 w605 w613 w617 w623 w632]
      tunnel: [w555 w559 w569 w577 w599 w604 w612 w617 w622 w631] -> w552
      tunnel: [FALSE FALSE ("Stop") FALSE ("Stop") FALSE ("Stop") FALSE ("Stop") FALSE ("Stop") w616 w618 FALSE ("Stop") FALSE ("Stop")] -> w550
      event Timeout {
        # "Timeout is executed when no other event is triggered."
        n190 = event-data() -> ()  [unwired: 1 in, 1 out]
      }
      event "Top Level Folder Path": Value Change {
        # "This event is triggered when there is a value change in the folder path control."
        n191 = event-data() -> ("NewVal"=w558:path)  [unwired: 1 in]
        n192 = To Variant(anything=w558) -> (Variant=w557:variant)
        n193 = Bundle By Name(cluster=T2 {"State"="", "Data"=variant} ("Dequeue Element"), "State"="Get Path", "Data"=w557) -> (w562:T2)
        n194 = Build Array(w562) -> (w561:T2[])
        n195 = call "FileExplorerQueueDriver.vi"("Enqueue N Element"=w561, "error in (no error)"=w560, "Enum"=FileExplorerQueueOperations."Enqueue N") -> ("error out"=w559:errorcluster)  [unwired: 11 in, 1 out]
      }
      event "Tree": event #0x1e {
        # "Thi event is triggered when tree drop down is pressed."
        n196 = event-data() -> ("Tag"=w568:string)  [unwired: 1 in]
        n197 = To Variant(anything=w568) -> (Variant=w567:variant)
        n198 = Bundle By Name(cluster=T2 {"State"="", "Data"=variant} ("Dequeue Element"), "State"="Checked Folder", "Data"=w567) -> (w572:T2)
        n199 = Build Array(w572) -> (w571:T2[])
        n200 = call "FileExplorerQueueDriver.vi"("Enqueue N Element"=w571, "error in (no error)"=w570, "Enum"=FileExplorerQueueOperations."Enqueue N") -> ("error out"=w569:errorcluster)  [unwired: 11 in, 1 out]
      }
      event "Tree": Item Close {
        # "Thi event is triggered when tree item is closed."
        n201 = event-data() -> ("Tag"=w576:string)  [unwired: 1 in]
        n202 = To Variant(anything=w576) -> (Variant=w579:variant)
        n203 = Bundle By Name(cluster=T2 {"State"="", "Data"=variant} ("Dequeue Element"), "State"="Uncheck Folder", "Data"=w579) -> (w581:T2)
        n204 = Build Array(w581) -> (w580:T2[])
        n205 = call "FileExplorerQueueDriver.vi"("Enqueue N Element"=w580, "error in (no error)"=w578, "Enum"=FileExplorerQueueOperations."Enqueue N") -> ("error out"=w577:errorcluster)  [unwired: 11 in, 1 out]
      }
      event "Tree": Mouse Down {
        # "Thiis event is triggered when the mouse is pressed down on any tree item."
        n206 = event-data() -> ("Coords"=w597:T4)  [unwired: 1 in, 3 out]
        n207 = invoke on="Tree" class="Tree (strict)" method="Point To Row Column"(error in=w600, "Point"=w597) -> (error out=w598:errorcluster, "Tag"=w589:string, "Col"=w596:i32)  [unwired: 6 in, 5 out]
        n208 = Number To Fractional String(number=w596, precision (6)=i16 0) -> (F-format string=w588:string)  [unwired: 2 in]
        n209 = Build Array(w589, w588) -> (w587:string[])
        n210 = To Variant(anything=w587) -> (Variant=w591:variant)
        n211 = Bundle By Name(cluster=T2 {"State"="", "Data"=variant} ("Dequeue Element"), "State"="Trigger Sort", "Data"=w591) -> (w592:T2)
        n212 = Build Array(w592) -> (w590:T2[])
        n213 = call "FileExplorerQueueDriver.vi"("Enqueue N Element"=w590, "error in (no error)"=w598, "Enum"=FileExplorerQueueOperations."Enqueue N") -> ("error out"=w599:errorcluster)  [unwired: 11 in, 1 out]
      }
      event "Copy": Value Change {
        # "Thi event is triggered when there is a value change in the copy boolean."
        n214 = event-data() -> ("NewVal"=w603:bool)  [unwired: 1 in]
        n215 = To Variant(anything=w603) -> (Variant=w611:variant)
        n216 = Bundle By Name(cluster=T2 {"State"="", "Data"=variant} ("Dequeue Element"), "State"="Copy", "Data"=w611) -> (w609:T2)
        n217 = Build Array(w609) -> (w610:T2[])
        n218 = call "FileExplorerQueueDriver.vi"("Enqueue N Element"=w610, "error in (no error)"=w605, "Enum"=FileExplorerQueueOperations."Enqueue N") -> ("error out"=w604:errorcluster)  [unwired: 11 in, 1 out]
      }
      event Panel Close? {
        w616 = TRUE ("Discard?")
        # "This event is triggered when the front panel is closed."
        n219 = event-data() -> ()  [unwired: 1 in, 2 out]
        n220 = call "FileExplorerQueueDriver.vi"("Enqueue Element"=T2 {"State"="Exit", "Data"=variant}, "error in (no error)"=w613, "Enum"=FileExplorerQueueOperations."Enqueue") -> ("error out"=w612:errorcluster)  [unwired: 11 in, 1 out]
        n221 = event-data("Discard?"=w616) -> ()  [unwired: 1 in, 1 out]
      }
      event User Event {
        # "This event stops this producer loop when stop user event is generated in the consumer loop."
        n222 = event-data() -> ("Stop"=w618:bool)  [unwired: 1 in]
      }
      event "Expand / Colapse": Value Change {
        # "Thi event is triggered when there is a value change in the collapse boolean."
        n223 = event-data() -> ("NewVal"=w627:bool)  [unwired: 1 in]
        n224 = To Variant(anything=w627) -> (Variant=w626:variant)
        n225 = Bundle By Name(cluster=T2 {"State"="", "Data"=variant} ("Dequeue Element"), "State"="Expand or ColapseTree", "Data"=w626) -> (w621:T2)
        n226 = Build Array(w621) -> (w620:T2[])
        n227 = call "FileExplorerQueueDriver.vi"("Enqueue N Element"=w620, "error in (no error)"=w623, "Enum"=FileExplorerQueueOperations."Enqueue N") -> ("error out"=w622:errorcluster)  [unwired: 11 in, 1 out]
      }
      event "Search Bar": Value Change {
        # "Thi event is triggered when there is a value change in the search bar- string control."
        n228 = event-data() -> ("NewVal"=w630:string)  [unwired: 1 in]
        n229 = To Variant(anything=w630) -> (Variant=w629:variant)
        n230 = Bundle By Name(cluster=T2 {"State"="", "Data"=variant} ("Dequeue Element"), "State"="Search File", "Data"=w629) -> (w634:T2)
        n231 = Build Array(w634) -> (w633:T2[])
        n232 = call "FileExplorerQueueDriver.vi"("Enqueue N Element"=w633, "error in (no error)"=w632, "Enum"=FileExplorerQueueOperations."Enqueue N") -> ("error out"=w631:errorcluster)  [unwired: 11 in, 1 out]
      }
    }
  }
  n233 = Unregister For Events(event registration refnum=w6, error in=w16) -> (error out=w7:errorcluster)
  n234 = Destroy User Event(user event=w3, error in=w7) -> (error out=w5:errorcluster)
  n235 = Merge Errors(w5, w17) -> (→"error out":errorcluster)
